vi "volumeCenter.vi"(0 "xyz order":bool, 1 "input array":u32[][][](array[numeric])) -> (4 "mean location":cluster{"x":dbl, "y":dbl, "z":dbl})   [LabVIEW 2010]
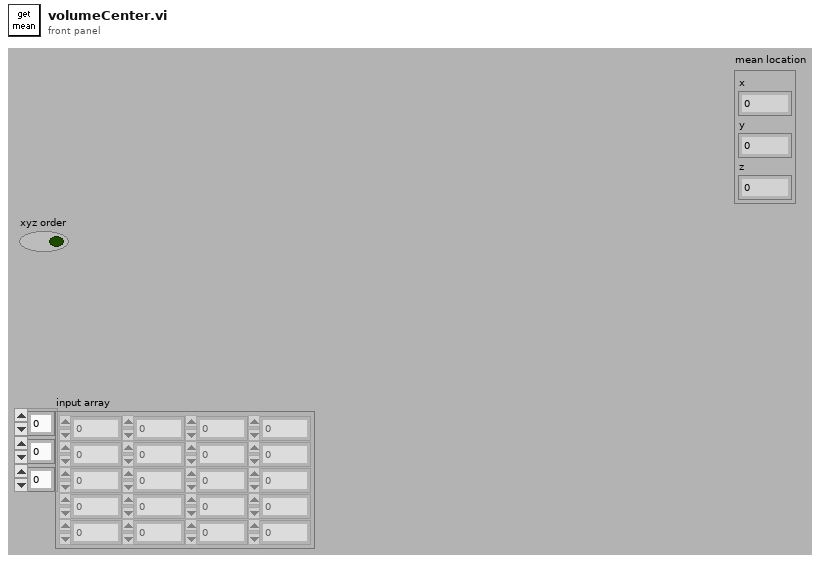
[diagram p1: front panel]
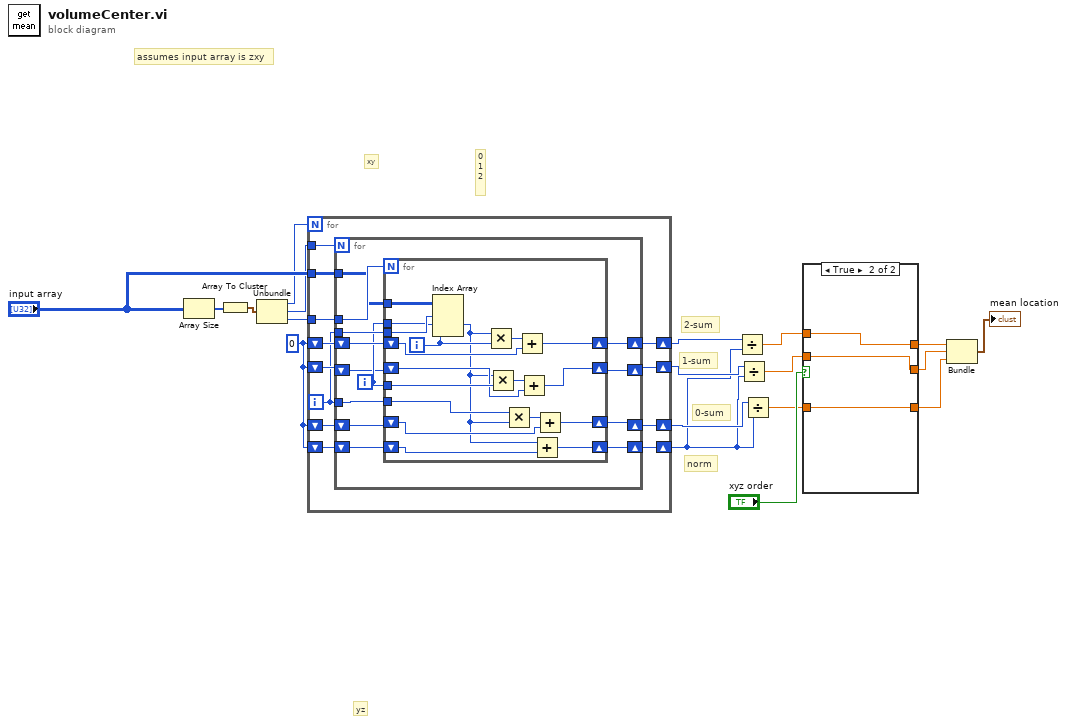
[diagram p0: block diagram]
diagram:
  w13 = u32 0
  # "0\n1\n2"
  # "norm"
  # "0-sum"
  # "1-sum"
  # "2-sum"
  # "yz"
  # "xy"
  # "assumes input array is zxy"
  n1 = Array Size(array="input array") -> (size(s)=w18:i32[])
  n2 = Array To Cluster(array=w18) -> (cluster=w17:cluster{"[0]":i32, "[1]":i32, "[2]":i32})
  n3 = Unbundle(w17) -> ("[0]"=w16:i32, "[1]"=w15:i32, "[2]"=w14:i32)
  n4 = for {
    N: w16 -> [_]
    tunnel: "input array" -> [w31]
    tunnel: w15 -> [w30]
    tunnel: w14 -> [w29]
    shift-right: [w28] -> w12
    shift-left: w13 -> [w27]
    shift-right: [w26] -> w11
    shift-left: w13 -> [w25]
    shift-right: [w23] -> w10
    shift-left: w13 -> [w22]
    shift-right: [w21] -> w9
    shift-left: w13 -> [w20]
    i -> [w24]
    n5 = for {
      N: w30 -> [_]
      tunnel: w31 -> [w43]
      tunnel: w24 -> [w42]
      tunnel: w29 -> [w44]
      shift-right: [w41] -> w28
      shift-left: w27 -> [w40]
      shift-right: [w38] -> w26
      shift-left: w25 -> [w37]
      tunnel: w24 -> [w36]
      shift-right: [w35] -> w23
      shift-left: w22 -> [w34]
      shift-right: [w33] -> w21
      shift-left: w20 -> [w32]
      i -> [w39]
      n6 = for {
        N: w44 -> [_]
        tunnel: w43 -> [w62]
        tunnel: w42 -> [w61]
        tunnel: w39 -> [w60]
        shift-right: [w57] -> w41
        shift-left: w40 -> [w56]
        tunnel: w39 -> [w54]
        shift-right: [w53] -> w38
        shift-left: w37 -> [w52]
        tunnel: w36 -> [w50]
        shift-right: [w49] -> w35
        shift-left: w34 -> [w48]
        shift-right: [w46] -> w33
        shift-left: w32 -> [w45]
        i -> [w59]
        n7 = Index Array(array=w62, index (dim 0)=w61, index (dim 1)=w60, index (dim 2)=w59) -> (element=w47:u32)
        n8 = Multiply(x=w47, y=w59) -> (x*y=w58:u32)
        n9 = Multiply(x=w47, y=w54) -> (x*y=w55:u32)
        n10 = Multiply(x=w50, y=w47) -> (x*y=w51:u32)
        n11 = Add(x=w58, y=w56) -> (x+y=w57:u32)
        n12 = Add(x=w55, y=w52) -> (x+y=w53:u32)
        n13 = Add(x=w47, y=w45) -> (x+y=w46:u32)
        n14 = Add(x=w51, y=w48) -> (x+y=w49:u32)
      }
    }
  }
  n15 = Divide(x=w12, y=w9) -> (x/y=w7:dbl)
  n16 = Divide(x=w11, y=w9) -> (x/y=w6:dbl)
  n17 = Divide(x=w10, y=w9) -> (x/y=w5:dbl)
  n18 = case shown="True" "xyz order" {
    tunnel: [w64 w68] -> w4
    tunnel: w7 -> [w63 w68]
    tunnel: [w65 w67] -> w3
    tunnel: w6 -> [w64 w67]
    tunnel: [w63 w66] -> w2
    tunnel: w5 -> [w65 w66]
    frame False {
    }
    frame True {
    }
  }
  n19 = Bundle(w4, w3, w2) -> (→"mean location":cluster{dbl, dbl, dbl})  [unwired: 1 in]
